vi "LS218_LIRE_CONFIG.vi"(8 "entrée d'erreur (pas d'erreur)":errorcluster) -> (0 "sortie d'erreur":errorcluster, 1 "PERIODE":i8, 2 "Voies de mesures":T1(array[cluster]), 3 "Celsius":bool, 4 "DOSSIER":path, 5 "value 2":i32 caption="T5_8", 6 "NOM MANIP":string, 7 "value":i32 caption="T1_4")   [LabVIEW 2016]
uses:
  <vilib>/Utility/config.llb/Read Key (Boolean).vi
  <vilib>/Utility/config.llb/Read Key (Path).vi
  <vilib>/Utility/config.llb/Read Key (String).vi
  <vilib>/Utility/config.llb/Read Key (I32).vi
  <vilib>/Utility/config.llb/NI_LVConfig.lvlib
panel:
  out "Numérique":i32
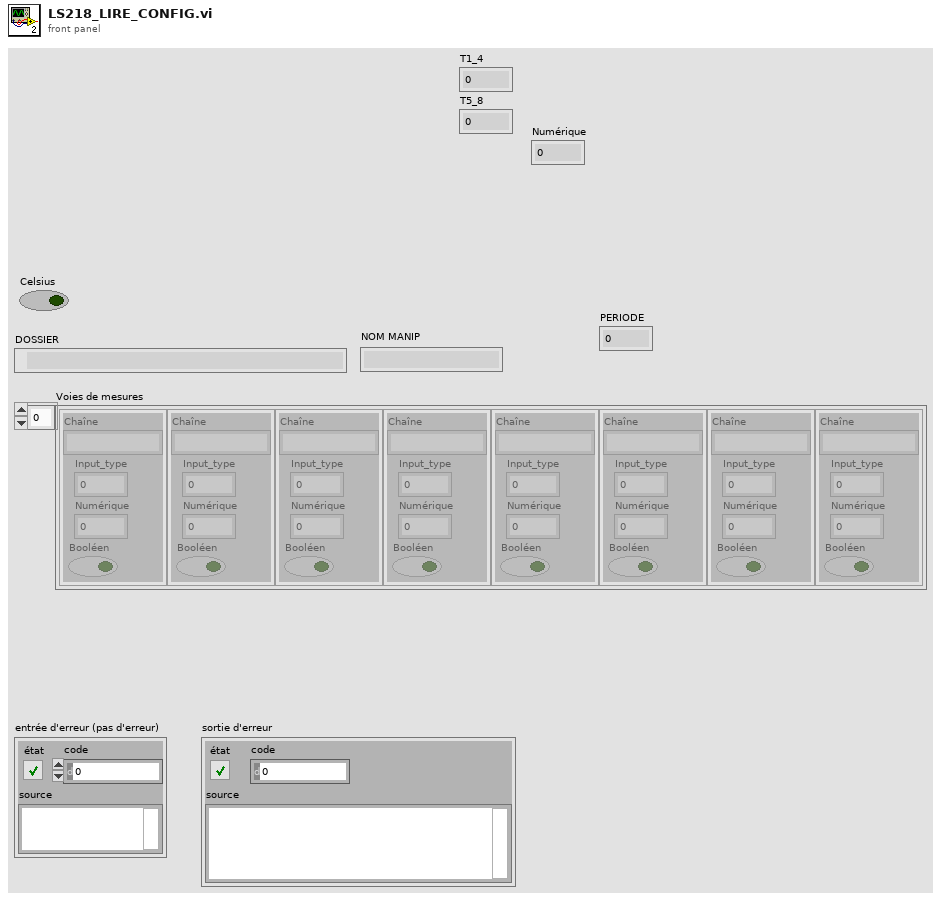
[diagram p1: front panel]
types:
  T1 = cluster{"Chaîne":string, "Input_type":u16, "Numérique":dbl, "Booléen":bool}[]
  T2 = typedef "NI_LVConfig.lvlib/Config Data RefNum.ctl" = refnum<k1>
  T3 = cluster{"Chaîne":string, "Input_type":u16, "Numérique":dbl, "Booléen":bool}
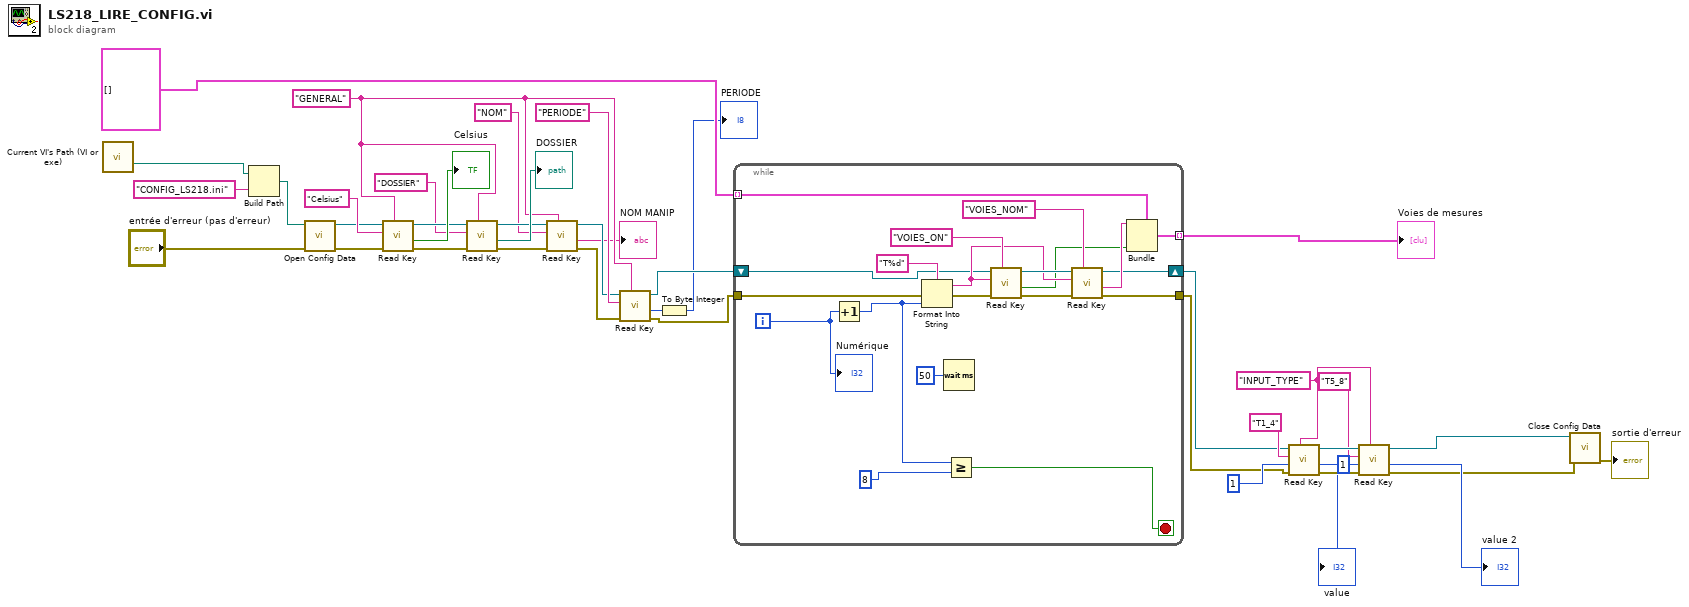
[diagram p0: block diagram]
diagram:
  w23 = "INPUT_TYPE" ("section")
  w3 = "GENERAL" ("section")
  n1 = call "Current VI's Path (VI or exe).vi"() -> ("VI or executable installation directory"=w29:path)  [unwired: 14 in, 1 out]
  n2 = Build Path(base path=w29, name or relative path="CONFIG_LS218.ini" ("nom ou chemin relatif")) -> (appended path=w28:path)
  n3 = call <vilib>:"Open Config Data.vi"("error in (no error)"="entrée d'erreur (pas d'erreur)", "configuration file path"=w28) -> ("error out"=w37:errorcluster, "refnum"=w38:T2)  [unwired: 7 in, 1 out]
  n4 = call-poly <vilib>:"Read Key.vi"("section"=w3, "error in (no error)"=w37, "key"="Celsius", "refnum"=w38) -> ("error out"=w35:errorcluster, "value"=→"Celsius":bool, "refnum out"=w34:T2)  [unwired: 4 in, 1 out]
  n5 = call-poly <vilib>:"Read Key.vi"("section"=w3, "error in (no error)"=w35, "key"="DOSSIER", "refnum"=w34) -> ("error out"=w7:errorcluster, "value"=→"DOSSIER":path, "refnum out"=w4:T2)  [unwired: 4 in, 1 out]
  n6 = call-poly <vilib>:"Read Key.vi"("section"=w3, "error in (no error)"=w7, "key"="NOM", "refnum"=w4) -> ("error out"=w6:errorcluster, "value"=→"NOM MANIP":string, "refnum out"=w5:T2)  [unwired: 4 in, 1 out]
  n7 = call-poly <vilib>:"Read Key.vi"("section"=w3, "error in (no error)"=w6, "key"="PERIODE", "refnum"=w5) -> ("error out"=w12:errorcluster, "value"=w9:i32, "refnum out"=w11:T2)  [unwired: 4 in, 1 out]
  n8 = To Byte Integer(number=w9) -> (8bit integer=→"PERIODE":i8)
  n9 = while {
    tunnel: [w60] -> w27 mode=indexing
    tunnel: T1 [] ("Voies de mesures") -> [w49] mode=indexing
    tunnel: [w47] -> w16
    tunnel: w12 -> [w46]
    shift-right: [w44] -> w15
    shift-left: w11 -> [w45]
    i -> [w50]
    stop <- w41 stop-if-true
    n10 = Increment(x=w50) -> (x+1=w43:i32)
    n11 = Format Into String(format string="T%d" ("key"), error in=w46, w43) -> (resulting string=w53:string, error out=w56:errorcluster)  [unwired: 1 in]
    n12 = Wait (ms)(milliseconds to wait=u32 50 ("attente (ms)")) -> ()  [unwired: 1 out]
    n13 = Greater Or Equal?(x=w43, y=8) -> (x >= y?=w41:bool)
    n14 = call-poly <vilib>:"Read Key.vi"("section"="VOIES_ON", "error in (no error)"=w56, "key"=w53, "refnum"=w45) -> ("error out"=w55:errorcluster, "value"=w51:bool, "refnum out"=w54:T2)  [unwired: 4 in, 1 out]
    n15 = call-poly <vilib>:"Read Key.vi"("section"="VOIES_NOM", "error in (no error)"=w55, "key"=w53, "refnum"=w54) -> ("error out"=w47:errorcluster, "value"=w52:string, "refnum out"=w44:T2)  [unwired: 4 in, 1 out]
    n16 = Bundle(cluster=w49, "Chaîne"=w52, "Booléen"=w51) -> (w60:T3)  [unwired: 2 in]
    "Numérique" <- w50
  }
  "Voies de mesures" <- w27
  n17 = call-poly <vilib>:"Read Key.vi"("section"=w23, "error in (no error)"=w16, "default value"=1, "key"="T1_4", "refnum"=w15) -> ("error out"=w25:errorcluster, "value"=→"value":i32, "refnum out"=w24:T2)  [unwired: 3 in, 1 out]
  n18 = call-poly <vilib>:"Read Key.vi"("section"=w23, "error in (no error)"=w25, "default value"=1, "key"="T5_8", "refnum"=w24) -> ("error out"=w13:errorcluster, "value"=→"value 2":i32, "refnum out"=w14:T2)  [unwired: 3 in, 1 out]
  n19 = call <vilib>:"Close Config Data.vi"("error in (no error)"=w13, "refnum"=w14) -> ("error out"=→"sortie d'erreur":errorcluster)  [unwired: 8 in, 1 out]
